vi "BuildErrStr.vi"(10 "ErrorIn":errorcluster, 11 "IinitString":string) -> (3 "OutMsg":string)   [LabVIEW 2015]
uses:
  <vilib>/Utility/error.llb/DialogType.ctl
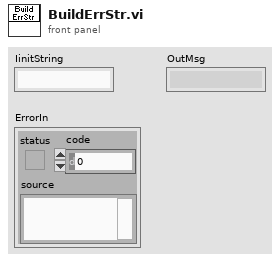
[diagram p1: front panel]
types:
  T1 = typedef "DialogType.ctl" = u16
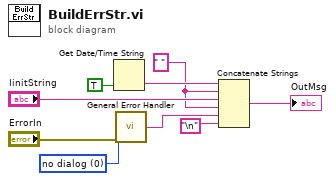
[diagram p0: block diagram]
diagram:
  w2 = T1 0 items=["no dialog", "OK message", "continue or stop message", "OK message + warnings", "continue/stop + warnings"] ("type of dialog (OK msg:1)")
  w3 = " "
  n1 = Get Date/Time String(want seconds? (F)=TRUE) -> (time string=w7:string)  [unwired: 2 in, 1 out]
  n2 = call <vilib>:"General Error Handler.vi"("type of dialog (OK msg:1)"=w2, "error in (no error)"="ErrorIn") -> ("source out"=w1:string)  [unwired: 9 in, 4 out]
  n3 = Concatenate Strings(w7, w3, "IinitString", w3, w1, "\n") -> (→"OutMsg":string)
